vi "NKTP_API_UnregUserEvents.vi"(7 "Event Registration Refnum":refnum<event-registration>, 8 "error in":errorcluster, 9 "Register Status User Event":refnum<user-event>, 10 "Device Status User Event":refnum<user-event>, 11 "Port Status User Event":refnum<user-event>) -> (0 "error out":errorcluster)   [LabVIEW 2015, in "NKTP_API.lvlib"]
doc: "Unregisters NKTP User Events. Unregistration of your own User Events can be added to this unregister VI."
uses:
  <instrlib>/NKTP_API/NKTP_API.lvlib
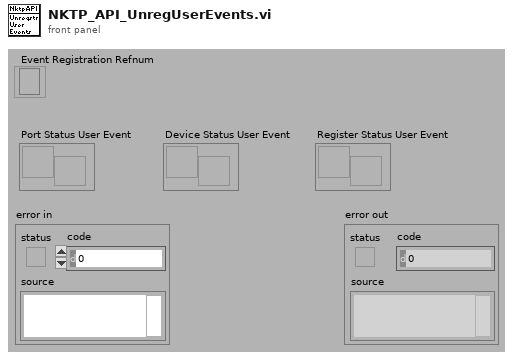
[diagram p1: front panel]
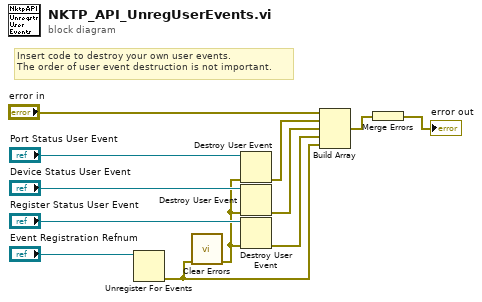
[diagram p0: block diagram]
diagram:
  # "Insert code to destroy your own user events.\nThe order of user event destruction is not important."
  n1 = Unregister For Events(event registration refnum="Event Registration Refnum") -> (error out=w2:errorcluster)  [unwired: 1 in]
  n2 = call <vilib>:"Clear Errors.vi"("error in (no error)"=w2) -> ("error out"=w7:errorcluster)  [unwired: 5 in, 1 out]
  n3 = Destroy User Event(user event="Port Status User Event", error in=w7) -> (error out=w5:errorcluster)
  n4 = Destroy User Event(user event="Device Status User Event", error in=w7) -> (error out=w4:errorcluster)
  n5 = Destroy User Event(user event="Register Status User Event", error in=w7) -> (error out=w3:errorcluster)
  n6 = Build Array("error in", w5, w4, w3, w2) -> (w1:errorcluster[])
  n7 = Merge Errors(w1) -> (→"error out":errorcluster)
